vi "Create Rectangle.vi"(8 "error in (no error)":errorcluster, 10 "Filled":bool) -> (0 "error out":errorcluster, 3 "Rectangle out":refnum<class "Rectangle.lvclass">)   [LabVIEW 2015, in "LV Image Editor Framework.lvlib" / "Rectangle.lvclass"]
uses:
  Rectangle.lvclass
  Rectangle.lvclass/Rectangle.ctl
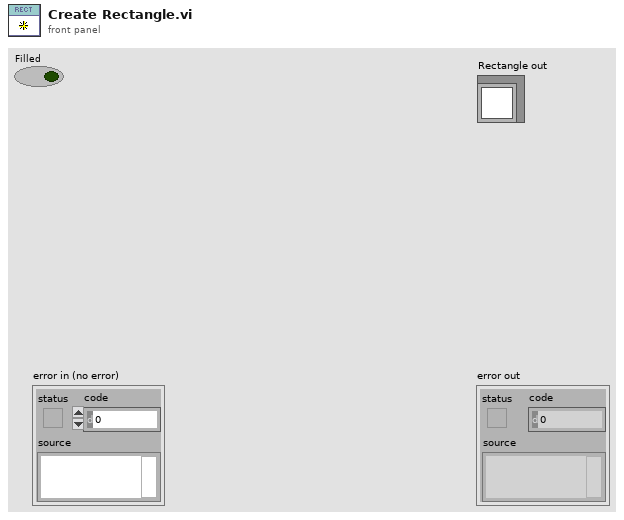
[diagram p1: front panel]
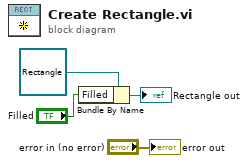
[diagram p0: block diagram]
diagram:
  n1 = Bundle By Name(cluster=refnum<class "Rectangle.lvclass"> refnum ("Rectangle in"), "Filled"="Filled") -> (→"Rectangle out":refnum<class "Rectangle.lvclass">)
  "error out" <- "error in (no error)"
